vi "BRig_dataCurrent_T_Cue_Audio_end.vi"() -> (2 "output_T_Cue_Audio_end":i32)   [LabVIEW 2014]
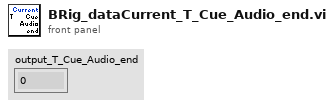
[diagram p1: front panel]
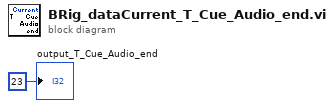
[diagram p0: block diagram]
diagram:
  "output_T_Cue_Audio_end" <- 23 ("output_iBlock")
